vi "Actor Core.vi"(8 "error in":errorcluster, 11 "UI Status in":refnum<class "UI Status.lvclass">) -> (0 "error out":errorcluster, 3 "Actor out":refnum<class "Actor.lvclass">)   [LabVIEW 2020, in "UI Status.lvlib" / "UI Status.lvclass"]
doc: "(<B>Filename</B>: Actor Framework.lvlib:Actor.lvclass:Actor Core.vi)\n\nReceives messages to the actor, reacts to them, and initiates any error handling that may shut the actor down.\n\nDescendant classes may override this VI to append parallel tasks for the actor to complete while it handles messages. Overrides use the Call Parent Class Method node."
uses:
  UI Status.lvclass
  Applications/National Instruments/LabVIEW 2020 64-bit/vi.lib/ActorFramework/Actor/Actor.lvclass
  <vilib>/ActorFramework/Actor/Actor.lvclass
  <vilib>/ActorFramework/Actor/Actor.lvclass/Actor.ctl
  <vilib>/ActorFramework/Message Enqueuer/Message Enqueuer.lvclass/Message Enqueuer.ctl
  UI Status.lvclass/UI Status.ctl
  RootActor/RootActor Messages/Load SubPanel Msg/Load SubPanel Msg.lvclass/Load SubPanel Msg.ctl
  <vilib>/ActorFramework/Message Enqueuer/Init from Existing Queue.vi
  <vilib>/ActorFramework/Message Enqueuer/Enqueue.vi
  <vilib>/ActorFramework/Stop Msg/Stop Msg.lvclass
  Applications/National Instruments/LabVIEW 2020 64-bit/vi.lib/ActorFramework/Message/Message.lvclass
  RootActor/RootActor Messages/Load SubPanel Msg/Load SubPanel Msg.lvclass
  <vilib>/ActorFramework/Message Priority Queue/Priority Enqueue.vi
  <vilib>/ActorFramework/Message Enqueuer/Message Enqueuer.lvclass
panel:
  out "Status":string
  out "TimeDate":string
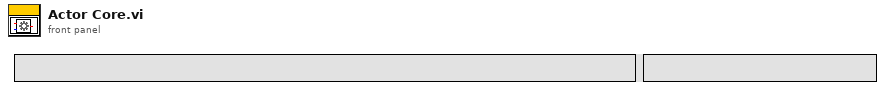
[diagram p1: front panel]
types:
  T1 = cluster{"Stop":refnum<user-event>, "Status":refnum<user-event>}
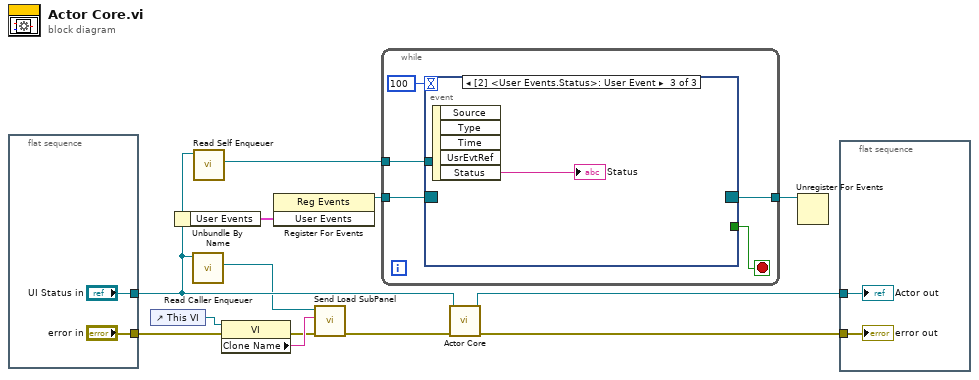
[diagram p0: block diagram]
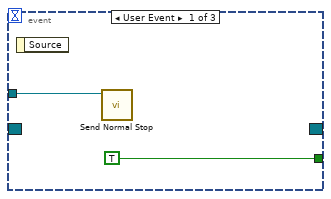
[diagram p2: hidden frame]
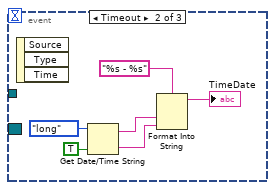
[diagram p3: hidden frame]
diagram:
  n1 = flat-sequence {
    tunnel: ["error in"] -> w2
    tunnel: ["UI Status in"] -> w6
    frame #0 {
    }
  }
  n2 = control-ref of="This VI"() -> (w7:refnum<vi>)
  n3 = Unbundle By Name(w6) -> ("User Events"=w11:T1)
  n4 = call <vilib>:"Read Caller Enqueuer.vi"("Actor"=w6) -> ("Caller Enqueuer"=w5:refnum<class "Message Enqueuer.lvclass">)  [unwired: 10 in]
  n5 = call <vilib>:"Read Self Enqueuer.vi"("Actor"=w6) -> ("Self Enqueuer"=w8:refnum<class "Message Enqueuer.lvclass">)  [unwired: 10 in]
  n6 = property class="VI"(reference=w7, error in=w2) -> (error out=w1:errorcluster, "Clone Name"=w3:string)  [unwired: 1 out]
  n7 = register-events(w11) -> (reference out=w10:refnum<event-registration>)  [unwired: 2 in, 1 out]
  n8 = call "Send Load SubPanel.vi"("error in (no error)"=w1, "Clone Name"=w3, "Message Enqueuer"=w5) -> ("error out"=w4:errorcluster)  [unwired: 7 in, 1 out]
  n9 = while {
    tunnel: w10 -> [w19]
    tunnel: [w18] -> w9
    tunnel: w8 -> [w17]
    stop <- w20 stop-if-true
    n10 = event shown="[2] <User Events.Status>: User Event" {
      selector: w19 -> [_ _ _]
      dyn-events: [_ _ _] -> w18
      timeout: 100 -> [_ _ _]
      tunnel: [TRUE _ _] -> w20
      tunnel: w17 -> [w21 _ _]
      event User Event {
        n11 = event-data() -> ()  [unwired: 1 in, 1 out]
        n12 = call <vilib>:"Send Normal Stop.vi"("Message Enqueuer"=w21) -> ()  [unwired: 10 in, 1 out]
      }
      event Timeout {
        n13 = event-data() -> ()  [unwired: 1 in, 3 out]
        n14 = Get Date/Time String(date format (0)=enum16{"short", "long", "abbreviated"}."long", want seconds? (F)=TRUE) -> (date string=w25:string, time string=w24:string)  [unwired: 1 in]
        n15 = Format Into String(format string="%s - %s", w25, w24) -> (resulting string=→"TimeDate":string)  [unwired: 2 in, 1 out]
      }
      event User Event {
        n16 = event-data() -> ("Status"=→"Status":string)  [unwired: 1 in, 4 out]
      }
    }
  }
  n17 = call-parent "Actor Core.vi"("error in"=w4, "Actor in"=w6) -> ("error out"=w13:errorcluster, "Actor out"=w12:refnum<class "Actor.lvclass">)  [unwired: 8 in]
  n18 = Unregister For Events(event registration refnum=w9) -> ()  [unwired: 1 in, 1 out]
  n19 = flat-sequence {
    tunnel: w13 -> [w31]
    tunnel: w12 -> [w30]
    frame #0 {
      "error out" <- w31
      "Actor out" <- w30
    }
  }
